vi "fgv_math-points.vi"(7 "cmd":T1, 11 "point-db":T2 {"wpt closest"."x" format="%.2f"; "wpt closest"."y" format="%.2f"; "center"."x" format="%.2f"; "center"."y" format="%.2f"; "lookahead circle in"."x" format="%.2f"; "lookahead circle in"."y" format="%.2f"; "looktail"."x" format="%.2f"; "looktail"."y" format="%.2f"; "lookahead"."x" format="%.2f"; "lookahead"."y" format="%.2f"}) -> (3 "point-db out":T2 {"wpt closest"."x" format="%.2f"; "wpt closest"."y" format="%.2f"; "center"."x" format="%.2f"; "center"."y" format="%.2f"; "lookahead circle in"."x" format="%.2f"; "lookahead circle in"."y" format="%.2f"; "looktail"."x" format="%.2f"; "looktail"."y" format="%.2f"; "lookahead"."x" format="%.2f"; "lookahead"."y" format="%.2f"})   [LabVIEW 2019]
uses:
  Ctrl/cmd_common.ctl
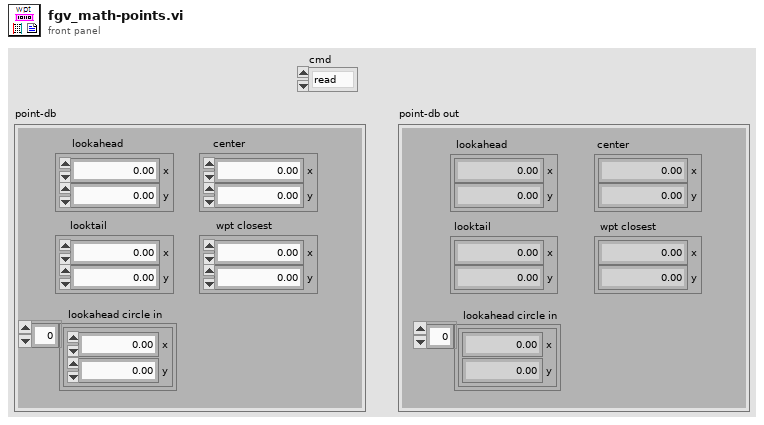
[diagram p1: front panel]
types:
  T1 = typedef "cmd_common.ctl" = enum16{"read", "write"}
  T2 = cluster{"lookahead":cluster{"x":dbl, "y":dbl}, "looktail":cluster{"x":dbl, "y":dbl}, "lookahead circle in":cluster{"x":dbl, "y":dbl}[], "center":cluster{"x":dbl, "y":dbl}, "wpt closest":cluster{"x":dbl, "y":dbl}}
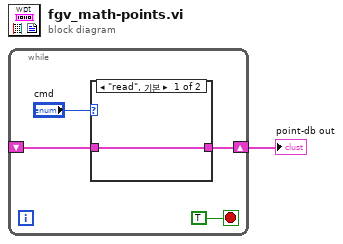
[diagram p0: block diagram]
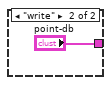
[diagram p2: hidden frame]
diagram:
  n1 = while {
    shift-right: [w3] -> w1
    shift-left: _ -> [w2]
    stop <- TRUE stop-if-true
    n2 = case shown="\"read\", 기본" "cmd" {
      tunnel: [w6 "point-db"] -> w3
      tunnel: w2 -> [w6 _]
      frame "read", Default {
      }
      frame "write" {
      }
    }
  }
  "point-db out" <- w1
